vi "GPS_parse.vi"(9 "GPS_Payload":u8[](array[numeric])=[131, 206, 19, 0, 0, 53, 149, 118, 0, 0] format="%.0x") -> (1 "PASS(T)":bool, 2 "Result":string, 3 "Distance":dbl format="%#_6f")   [LabVIEW 2024, in "Test_2.lvlib"]
uses:
  Test_2.lvlib
  <vilib>/Instr/_visa.llb/VISA Configure Serial Port (Instr).vi
  Launcher/Launcher_DTU.lvlib
panel:
  out "long":dbl
  out "lat":dbl
  out "String 2":string
  out "string 2":string
  out "String":string
  out "string":string
  out "f":string[](array[string])
  out "x/y":u32
  out "concatenated string":string
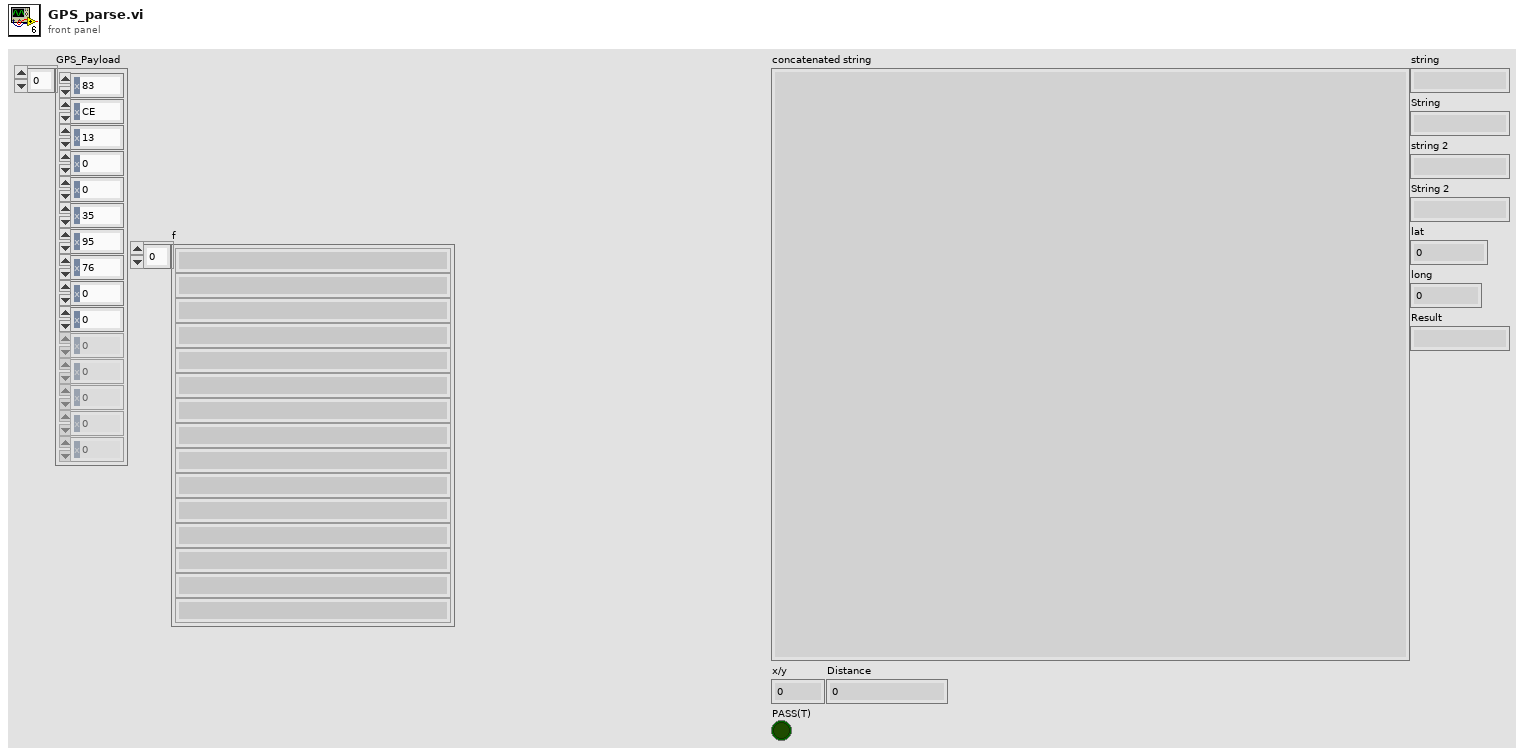
[diagram p1: front panel]
types:
  T1 = enum16{"Read", "Write", "All_sections", "All_values", "Remove key&section"}
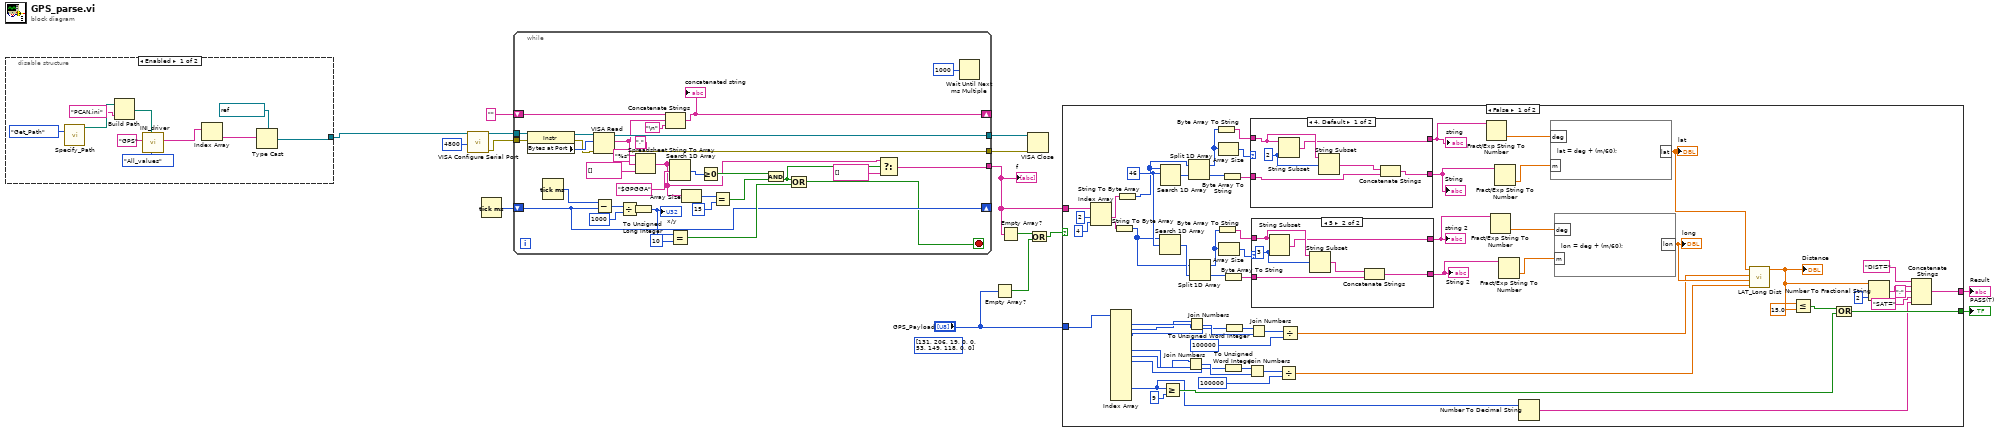
[diagram p0: block diagram]
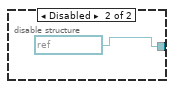
[diagram p2: hidden frame]
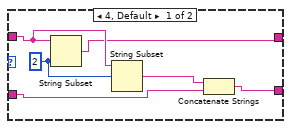
[diagram p3: hidden frame]
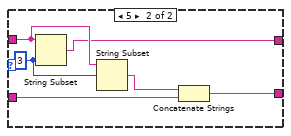
[diagram p4: hidden frame]
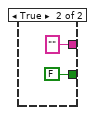
[diagram p5: hidden frame]
diagram:
  (unwired) u8[] [131, 206, 19, 0, 0, 53, 149, 118, 0, 0] ("GPS_Payload")
  n1 = disable-structure shown="Enabled" {
    disable-tunnel: [w16 refnum<visa-resource-name> "COM25" ("VISA resource name")] -> w6
    frame Enabled {
      n2 = call "Specify_Path.vi"("Path_Enum"=enum16{"Find_Path", "Get_Path"}."Get_Path") -> ("Configurations"=w24:path)  [unwired: 7 in, 7 out]
      n3 = Build Path(base path=w24, name or relative path="PCAN.ini") -> (appended path=w22:path)
      n4 = call "INI_driver.vi"("Enum"=T1."All_values", "instrument file path"=w22, "Section"="GPS") -> ("Values out"=w19:string[])  [unwired: 5 in, 3 out]
      n5 = Index Array(array=w19) -> (element=w18:string)  [unwired: 1 in]
      n6 = Type Cast(type=refnum<visa-resource-name> "COM26" ("VISA resource name"), x=w18) -> (*(type *) &x=w16:refnum<visa-resource-name>)
    }
    frame Disabled {
    }
  }
  n7 = call-poly "VISA Configure Serial Port"("VISA resource name"=w6, "baud rate (9600)"=u32 4800) -> ("VISA resource name out"=w14:refnum<visa-resource-name>, "error out"=w13:errorcluster)  [unwired: 12 in]
  n8 = Tick Count (ms)() -> (millisecond timer value=w9:u32)
  n9 = while {
    tunnel: w14 -> [w58]
    tunnel: w13 -> [w57]
    tunnel: [w56] -> w11
    tunnel: [w55] -> w12
    shift-right: [w53] -> _
    shift-left: "" -> [w54]
    shift-right: [w36] -> _
    shift-left: w9 -> [w36]
    tunnel: [w28] -> w7
    stop <- w32 stop-if-true
    n10 = property class="Instr"(reference=w58, error in=w57) -> (reference out=w60:refnum<visa-resource-name>, error out=w27:errorcluster, "Bytes at Port"=w59:u32)
    n11 = Tick Count (ms)() -> (millisecond timer value=w42:u32)
    n12 = VISA Read(VISA resource name=w60, byte count=w59, error in (no error)=w27) -> (VISA resource name out=w56:refnum<visa-resource-name>, read buffer=w34:string, error out=w55:errorcluster)  [unwired: 1 out]
    n13 = Subtract(x=w42, y=w36) -> (x-y=w41:u32)
    n14 = Divide(x=w41, y=u32 1000) -> (x/y=w39:dbl)
    n15 = To Unsigned Long Integer(number=w39) -> (unsigned 32bit integer=w33:u32)
    "x/y" <- w33
    n16 = Spreadsheet String To Array(delimiter (Tab)=",", format string="%s", spreadsheet string=w34, array type (2D Dbl)=string[] []) -> (array=w30:string[])
    n17 = Concatenate Strings(w54, w34, "\n") -> (w53:string)
    "concatenated string" <- w53
    n18 = Search 1D Array(1D array=w30, element="$GPGGA") -> (index of element=w46:i32)  [unwired: 1 in]
    n19 = Equal?(x=w33, y=u32 10) -> (x = y?=w37:bool)
    n20 = Array Size(array=w30) -> (size(s)=w45:i32)
    n21 = Greater Or Equal To 0?(x=w46) -> (x >= 0?=w35:bool)
    n22 = Equal?(x=w45, y=15) -> (x = y?=w43:bool)
    n23 = And(x=w35, y=w43) -> (x .and. y?=w31:bool)
    n24 = Compound Arithmetic op=OR(w31, w37) -> (w32:bool)
    n25 = Select(t=w30, s=w31, f=string[] []) -> (s? t:f=w28:string[])
    n26 = Wait Until Next ms Multiple(millisecond multiple=u32 1000) -> ()  [unwired: 1 out]
  }
  "f" <- w7
  n27 = Empty Array?(array="GPS_Payload") -> (empty?=w1:bool)
  n28 = Empty Array?(array=w7) -> (empty?=w8:bool)
  n29 = VISA Close(VISA resource name=w11, error in (no error)=w12) -> ()  [unwired: 1 out]
  n30 = Or(x=w8, y=w1) -> (x .or. y?=w3:bool)
  n31 = case shown="False" w3 {
    tunnel: w7 -> [w121 _]
    tunnel: "GPS_Payload" -> [w83 _]
    tunnel: [w70 FALSE] -> w5
    tunnel: [w61 ""] -> w4
    frame False {
      w116 = 46
      n32 = Index Array(array=w121, index #1=2 ("index"), index #2=4 ("index")) -> (element #1=w118:string, element #2=w117:string)
      n33 = Index Array(array=w83) -> (element #1=w82:u8, element #2=w81:u8, element #3=w80:u8, element #6=w79:u8, element #7=w78:u8, element #8=w77:u8, element #13=w62:u8)  [unwired: 15 in, 8 out]
      n34 = String To Byte Array(string=w117) -> (unsigned byte array=w102:u8[])
      n35 = String To Byte Array(string=w118) -> (unsigned byte array=w110:u8[])
      n36 = Search 1D Array(1D array=w102, element=w116) -> (index of element=w103:i32)  [unwired: 1 in]
      n37 = Search 1D Array(1D array=w110, element=w116) -> (index of element=w115:i32)  [unwired: 1 in]
      n38 = Greater Or Equal?(x=w62, y=u8 9 ("element")) -> (x >= y?=w71:bool)
      n39 = Join Numbers(hi=w78, lo=w79) -> ((hi.lo)=w87:u16)
      n40 = Join Numbers(hi=w81, lo=w82) -> ((hi.lo)=w91:u16)
      n41 = Split 1D Array(array=w110, index=w115) -> (first subarray=w113:u8[], second subarray=w111:u8[])
      n42 = Split 1D Array(array=w102, index=w103) -> (first subarray=w105:u8[], second subarray=w107:u8[])
      n43 = Byte Array To String(unsigned byte array=w113) -> (string=w112:string)
      n44 = Byte Array To String(unsigned byte array=w105) -> (string=w106:string)
      n45 = Array Size(array=w113) -> (size(s)=w114:i32)
      n46 = Array Size(array=w105) -> (size(s)=w104:i32)
      n47 = Byte Array To String(unsigned byte array=w111) -> (string=w109:string)
      n48 = Byte Array To String(unsigned byte array=w107) -> (string=w108:string)
      n49 = To Unsigned Word Integer(number=w77) -> (unsigned 16bit integer=w85:u16)
      n50 = To Unsigned Word Integer(number=w80) -> (unsigned 16bit integer=w89:u16)
      n51 = Join Numbers(hi=w85, lo=w87) -> ((hi.lo)=w84:u32)
      n52 = Join Numbers(hi=w89, lo=w91) -> ((hi.lo)=w88:u32)
      n53 = case shown="4, Default" w114 {
        tunnel: w112 -> [w138 w144]
        tunnel: [w134 w143] -> w101
        tunnel: w109 -> [w136 w141]
        tunnel: [w135 w140] -> w99
        frame 4, Default {
          w139 = 2 ("length (rest)")
          n54 = String Subset(string=w138, length (rest)=w139) -> (substring=w134:string)  [unwired: 1 in]
          n55 = String Subset(string=w138, offset (0)=w139) -> (substring=w137:string)  [unwired: 1 in]
          n56 = Concatenate Strings(w137, w136) -> (w135:string)
        }
        frame 5 {
          w145 = 3 ("length (rest)")
          n57 = String Subset(string=w144, length (rest)=w145) -> (substring=w143:string)  [unwired: 1 in]
          n58 = String Subset(string=w144, offset (0)=w145) -> (substring=w142:string)  [unwired: 1 in]
          n59 = Concatenate Strings(w142, w141) -> (w140:string)
        }
      }
      "string" <- w101
      "String" <- w99
      n60 = case shown="5" w104 {
        tunnel: w106 -> [w126 w132]
        tunnel: [w122 w131] -> w95
        tunnel: w108 -> [w124 w129]
        tunnel: [w123 w128] -> w94
        frame 4, Default {
          w127 = 2 ("length (rest)")
          n61 = String Subset(string=w126, length (rest)=w127) -> (substring=w122:string)  [unwired: 1 in]
          n62 = String Subset(string=w126, offset (0)=w127) -> (substring=w125:string)  [unwired: 1 in]
          n63 = Concatenate Strings(w125, w124) -> (w123:string)
        }
        frame 5 {
          w133 = 3 ("length (rest)")
          n64 = String Subset(string=w132, length (rest)=w133) -> (substring=w131:string)  [unwired: 1 in]
          n65 = String Subset(string=w132, offset (0)=w133) -> (substring=w130:string)  [unwired: 1 in]
          n66 = Concatenate Strings(w130, w129) -> (w128:string)
        }
      }
      "string 2" <- w95
      "String 2" <- w94
      n67 = Divide(x=w84, y=u64 100000) -> (x/y=w75:dbl)
      n68 = Divide(x=w88, y=u64 100000) -> (x/y=w76:dbl)
      n69 = Fract/Exp String To Number(string=w101) -> (number=w100:dbl)  [unwired: 3 in, 1 out]
      n70 = Fract/Exp String To Number(string=w95) -> (number=w96:dbl)  [unwired: 3 in, 1 out]
      n71 = Fract/Exp String To Number(string=w99) -> (number=w98:dbl)  [unwired: 3 in, 1 out]
      n72 = Fract/Exp String To Number(string=w94) -> (number=w97:dbl)  [unwired: 3 in, 1 out]
      n73 = Number To Decimal String(number=w62) -> (decimal integer string=w63:string)  [unwired: 1 in]
      n74 = formula code="lat = deg + (m/60);"("deg"=w100, "m"=w98) -> ("lat"=w93:dbl)
      "lat" <- w93
      n75 = formula code="lon = deg + (m/60);"("deg"=w96, "m"=w97) -> ("lon"=w92:dbl)
      "long" <- w92
      n76 = call "LAT_Long Dist.vi"("long_DTU"=w75, "long"=w92, "lat_DTU"=w76, "lat"=w93) -> ("Distance"=w68:dbl)  [unwired: 7 in]
      "Distance" <- w68
      n77 = Less Or Equal?(x=w68, y=15.0) -> (x <= y?=w72:bool)
      n78 = Compound Arithmetic op=OR(w72, w71) -> (w70:bool)
      n79 = Number To Fractional String(number=w68, precision (6)=i16 2) -> (F-format string=w66:string)  [unwired: 2 in]
      n80 = Concatenate Strings("DIST=", w66, ";" ("string"), "SAT=" ("string"), w63) -> (w61:string)
    }
    frame True {
    }
  }
  "PASS(T)" <- w5
  "Result" <- w4
